vi "Write configuration.vi"(8 "error in (no error)":errorcluster, 11 "focus in":refnum<class "focus.lvclass">) -> (0 "error out":errorcluster, 3 "focus out":refnum<class "focus.lvclass">)   [LabVIEW 2012, in "focus.lvclass"]
doc: "Writes the configuration cluster into the configuration file. Configuration file is XML-based. It's name is <component ID>.xml"
uses:
  focus.lvclass
  <vilib>/Distrio/Murmex/Murmex/Murmex.lvclass
  focus.lvclass/focus.ctl
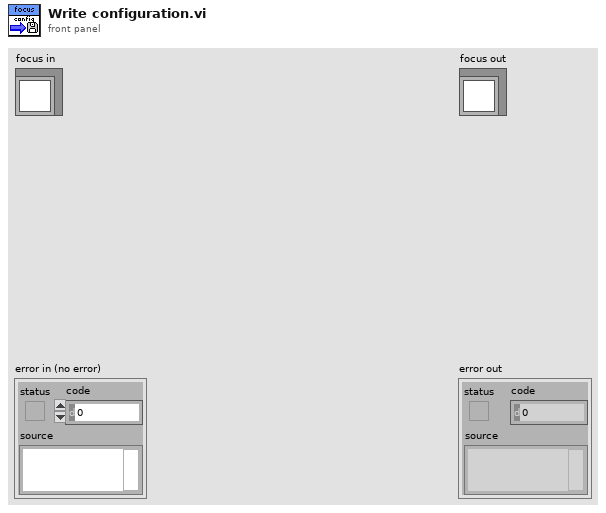
[diagram p1: front panel]
types:
  T1 = typedef "focus.lvclass/configuration_cluster.ctl" = cluster{"Port":T2, "Baudrate":T3, "update frequency":dbl[unit], "S/N Master controller":string, "Interface":T4, "soft limit min":dbl, "soft limit max":dbl, "startup speed":dbl[unit]}
  T2 = typedef "focus.lvclass/port_focus.ctl" = i32
  T3 = typedef "focus.lvclass/baud_rate_focus.ctl" = u16
  T4 = typedef "focus.lvclass/connection_type_focus.ctl" = enum16{"RS232", "RS232 DaisyChain", "USB", "USB_DaisyChain"}
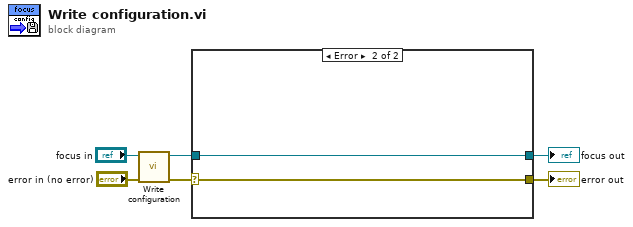
[diagram p0: block diagram]
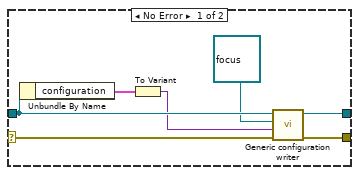
[diagram p2: hidden frame]
diagram:
  n1 = call-parent "Write configuration.vi"("error in (no error)"="error in (no error)", "Murmex in"="focus in") -> ("error out"=w4:errorcluster, "Murmex out"=w2:refnum<class "focus.lvclass">)  [unwired: 8 in]
  n2 = case shown="Error" w4 {
    selector: w4 -> [w13 w14]
    tunnel: [w12 w14] -> w3
    tunnel: w2 -> [w11 w15]
    tunnel: [w7 w15] -> w1
    frame No Error {
      n3 = Unbundle By Name(w11) -> ("configuration"=w10:T1)
      n4 = To Variant(anything=w10) -> (Variant=w8:variant)
      n5 = call <vilib>:"Generic configuration writer.vi"("error in (no error)"=w13, "configuration"=w8, "inheritance level"=refnum<class "focus.lvclass"> refnum ("focus"), "MurmexBase in"=w11) -> ("error out"=w12:errorcluster, "MurmexBase out"=w7:refnum<class "focus.lvclass">)  [unwired: 6 in]
    }
    frame Error {
    }
  }
  "error out" <- w3
  "focus out" <- w1
